vi "WiFi HttpUpload_Camera.vi"   [LabVIEW 2014]
uses:
  QwaveSys_ESP8266/QwaveSys_ESP8266.lvlib
  QwaveSys_Interface/QwaveSys_Interface.lvlib
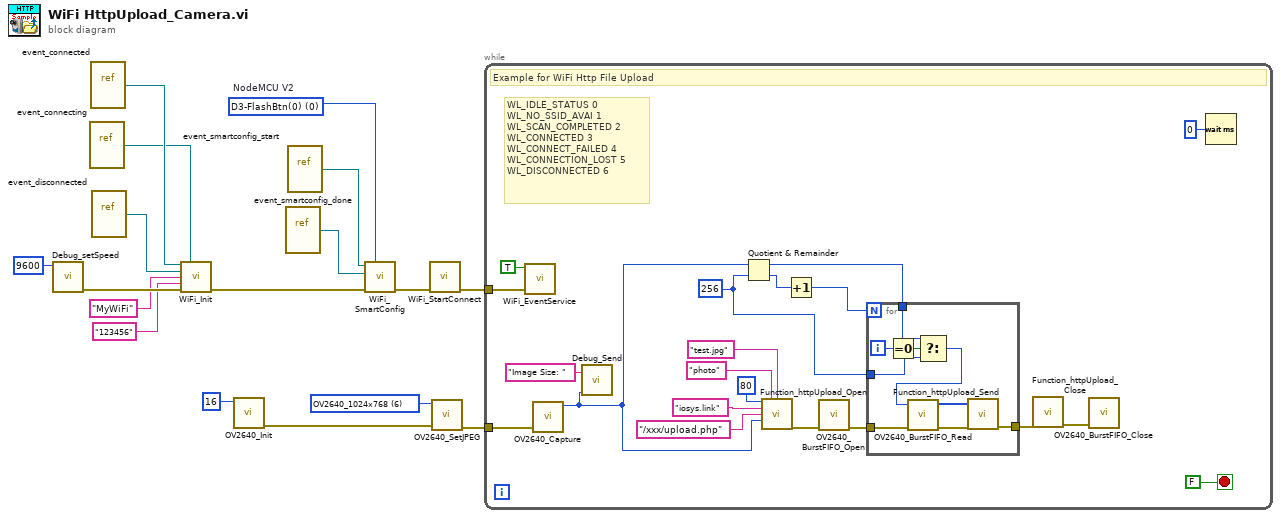
[diagram p0: block diagram]
diagram:
  w3 = u16 6 items=["OV2640_160x120", "OV2640_176x144", "OV2640_320x240", "OV2640_352x288", "OV2640_640x480", "OV2640_800x600", "OV2640_1024x768", "OV2640_1280x1024", "OV2640_1600x1200"] ("resolution")
  w10 = u8 0 items=["D0-(LED)-(16)"=16, "D1-SCL(5)"=5, "D2-SDA(4)"=4, "D3-FlashBtn(0)"=0, "D4-(2)"=2, "D5-SCK(14)"=14, "D6-MISO(12)"=12, "D7-MOSI(13)"=13, "D8-SS(15)"=15, "D9-TX(3)"=3, "D10-RX(1)"=1, "ADC0,(17)"=17]  # NodeMCU V2
  n1 = call "Debug_setSpeed.vi"("Speed"=u32 9600) -> ("error out"=w12:errorcluster)  [unwired: 10 in]
  n2 = vi-ref "event_connecting.vi"() -> (w7:refnum<vi>)
  n3 = vi-ref "event_connected.vi"() -> (w8:refnum<vi>)
  n4 = vi-ref "event_disconnected.vi"() -> (w6:refnum<vi>)
  n5 = call "WiFi_Init.vi"("connected"=w8, "connecting"=w7, "disconnected"=w6, "SSID"="MyWiFi", "PASSPHARSE"="123456", "error in (no error)"=w12) -> ("error out"=w17:errorcluster)  [unwired: 9 in]
  n6 = call "OV2640_Init.vi"("CS"=u8 16) -> ("error out"=w2:errorcluster)  [unwired: 9 in, 1 out]
  n7 = vi-ref "event_smartconfig_done.vi"() -> (w13:refnum<vi>)
  n8 = vi-ref "event_smartconfig_start.vi"() -> (w14:refnum<vi>)
  n9 = call "WiFi_SmartConfig.vi"("Smart Config Enter Pin"=w10, "error in (no error)"=w17, "smartconfig_done"=w13, "smartconfig_start"=w14) -> ("error out"=w16:errorcluster)  [unwired: 7 in]
  n10 = call "WiFi_StartConnect.vi"("error in (no error)"=w16) -> ("error out"=w15:errorcluster)  [unwired: 10 in]
  n11 = call "OV2640_SetJPEG.vi"("error in (no error)"=w2, "resolution"=w3) -> ("error out"=w1:errorcluster)  [unwired: 9 in]
  n12 = while {
    tunnel: w15 -> [w36]
    tunnel: w1 -> [w33]
    stop <- FALSE stop-if-true
    w21 = u32 256 ("y")
    # "WL_IDLE_STATUS\t0\nWL_NO_SSID_AVAI\t1\nWL_SCAN_COMPLETED\t2\nWL_CONNECTED\t3\nWL_CONNECT_FAILED\t4\nWL_CONNECTION_LOST\t5\nWL_DISCONNECTED\t6"
    # "Example for WiFi Http File Upload"
    n13 = call "WiFi_EventService.vi"("error in (no error)"=w36, "wait for connected (True)"=TRUE) -> ()  [unwired: 8 in, 2 out]
    n14 = call "OV2640_Capture.vi"("error in (no error)"=w33) -> ("FIFO Length"=w19:u32)  [unwired: 9 in, 1 out]
    n15 = call "Debug_Send.vi"("Name"="Image Size: ", "DATA"=w19) -> ()  [unwired: 10 in]
    n16 = Quotient & Remainder(x=w19, y=w21) -> (x-y*floor(x/y)=w22:u32, floor(x/y)=w26:u32)
    n17 = call "Function_httpUpload_Open.vi"("Port"=i8 80, "Name"="photo", "Filename"="test.jpg", "Host"="iosys.link", "URI"="/xxx/upload.php", "Upload Lenght"=w19) -> ("error out"=w28:errorcluster)  [unwired: 9 in]
    n18 = Increment(x=w26) -> (x+1=w23:u32)
    n19 = call "OV2640_BurstFIFO_Open.vi"("error in (no error)"=w28) -> ("error out"=w25:errorcluster)  [unwired: 10 in]
    n20 = for {
      N: w23 -> [_]
      tunnel: w25 -> [w44]
      tunnel: [w43] -> w24
      tunnel: w22 -> [w40]
      tunnel: w21 -> [w39]
      i -> [w42]
      n21 = Equal To 0?(x=w42) -> (x = 0?=w41:bool)
      n22 = Select(t=w40, s=w41, f=w39) -> (s? t:f=w38:u32)
      n23 = call "OV2640_BurstFIFO_Read.vi"("error in (no error)"=w44, "Lenght"=w38) -> ("error out"=w46:errorcluster, "DATA"=w45:u8[])  [unwired: 8 in]
      n24 = call "Function_httpUpload_Send.vi"("error in (no error)"=w46, "DATA"=w45) -> ("error out"=w43:errorcluster)  [unwired: 9 in]
    }
    n25 = call "Function_httpUpload_Close.vi"("error in (no error)"=w24) -> ("error out"=w27:errorcluster)  [unwired: 10 in]
    n26 = call "OV2640_BurstFIFO_Close.vi"("error in (no error)"=w27) -> ()  [unwired: 10 in, 1 out]
    n27 = Wait (ms)(milliseconds to wait=u32 0) -> ()  [unwired: 1 out]
  }
